vi "dfd_Lattice ARMA Normalization (OneM).vi"(7 "scale type":T1, 9 "coefficients v":dbl[](array[numeric]) format="%.2f", 10 "coefficients k":dbl[](array[numeric]) format="%.2f", 11 "x":dbl[](array[numeric])) -> (2 "norm":dbl[](array[numeric]) format="%.2f", 3 "y":dbl[](array[numeric]))   [LabVIEW 2017, in "NI_DigFilter_FXP.lvlib"]
uses:
  <vilib>/addons/Digital Filter Design/NI_DigFilter_FXP.lvlib
  <vilib>/addons/Digital Filter Design/_Objects.llb/DFD Coef Norm Type.ctl
  <vilib>/addons/Digital Filter Design/NI_DigFilterLicensed.lvlib
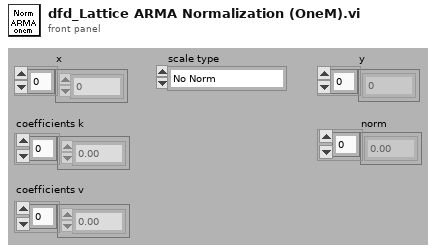
[diagram p1: front panel]
types:
  T1 = typedef "NI_DigFilterLicensed.lvlib/DFD Coef Norm Type.ctl" = enum16{"No Norm", "Time Domain 1-Norm", "Time Domain 2-Norm", "Time Domain Inf-Norm"}
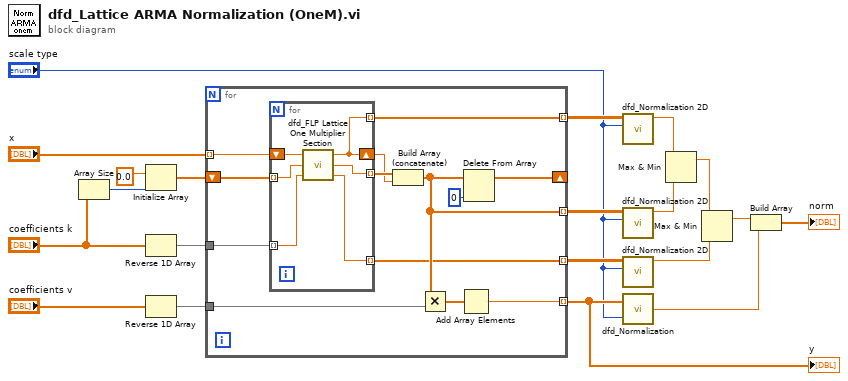
[diagram p0: block diagram]
diagram:
  n1 = Array Size(array="coefficients k") -> (size(s)=w19:i32)
  n2 = Initialize Array(0.0 ("element"), w19) -> (w20:dbl[])
  n3 = Reverse 1D Array(array="coefficients k") -> (reversed array=w18:dbl[])
  n4 = Reverse 1D Array(array="coefficients v") -> (reversed array=w17:dbl[])
  n5 = for {
    tunnel: w18 -> [w33]
    shift-right: [w28] -> _
    shift-left: w20 -> [w32]
    tunnel: [w22] -> w7 mode=indexing
    tunnel: w17 -> [w27]
    tunnel: [w26] -> w11 mode=indexing
    tunnel: [w25] -> w10 mode=indexing
    tunnel: "x" -> [w24] mode=indexing
    tunnel: [w21] -> w5 mode=indexing
    n6 = for {
      shift-right: [w36] -> w30
      shift-left: w24 -> [w39]
      tunnel: w32 -> [w38] mode=indexing
      tunnel: w33 -> [w37] mode=indexing
      tunnel: [w35] -> w31 mode=indexing
      tunnel: [w36] -> w26 mode=indexing
      tunnel: [w34] -> w21 mode=indexing
      n7 = call <vilib>:"dfd_FLP Lattice One Multiplier Section.vi"("k(m)"=w37, "w(m-1)"=w38, "x(m)"=w39) -> ("u(m)"=w34:dbl, "w(m)"=w35:dbl, "x(m-1)"=w36:dbl)
    }
    n8 = Build Array (concatenate)(w31, w30) -> (w25:dbl[])
    n9 = Multiply(x=w25, y=w27) -> (x*y=w23:dbl[])
    n10 = Add Array Elements(numeric array=w23) -> (sum=w22:dbl)
    n11 = Delete From Array(array=w25, index=0) -> (array with subset deleted=w28:dbl[])  [unwired: 1 in, 1 out]
  }
  "y" <- w7
  n12 = call <vilib>:"dfd_Normalization 2D.vi"("scale type"="scale type", "2D Array (col-major)"=w11) -> ("max norm"=w9:dbl)  [unwired: 9 out]
  n13 = call <vilib>:"dfd_Normalization 2D.vi"("scale type"="scale type", "2D Array (col-major)"=w10) -> ("max norm"=w8:dbl)  [unwired: 9 out]
  n14 = call <vilib>:"dfd_Normalization 2D.vi"("scale type"="scale type", "2D Array (col-major)"=w5) -> ("max norm"=w3:dbl)  [unwired: 9 out]
  n15 = call <vilib>:"dfd_Normalization.vi"("scale type"="scale type", "h(n)"=w7) -> ("norm"=w14:dbl)
  n16 = Max & Min(x=w9, y=w8) -> (max(x,y)=w2:dbl)  [unwired: 1 out]
  n17 = Max & Min(x=w2, y=w3) -> (max(x,y)=w1:dbl)  [unwired: 1 out]
  n18 = Build Array(w1, w14) -> (→"norm":dbl[])
